vi "Init Queue.vi"(8 "error in (no error)":errorcluster) -> (0 "error out":errorcluster, 3 "Queue out":refnum<queue>)   [LabVIEW 2017]
uses:
  Type Defs/Message.ctl
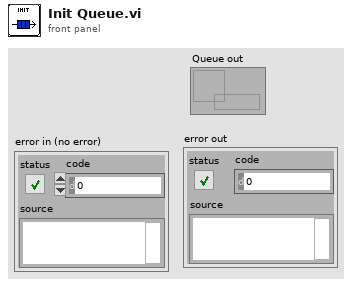
[diagram p1: front panel]
types:
  T1 = typedef "Message.ctl" = cluster{"State":string, "Message":variant}
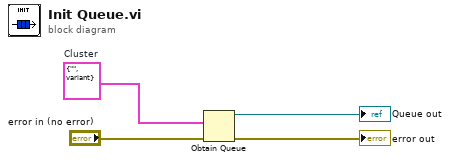
[diagram p0: block diagram]
diagram:
  w1 = T1 {"State"="", "Message"=variant}  # Cluster
  n1 = Obtain Queue(element data type=w1, error in (no error)="error in (no error)") -> (queue out=→"Queue out":refnum<queue>, error out=→"error out":errorcluster)  [unwired: 3 in, 1 out]
